vi "Cockpit_UDP_ receiver_IRISS_v2(2arms).vi"() -> ()   [LabVIEW 2016]
panel:
  in  "stop 2":bool
  out "deltaX 2":sgl
  out "data out 2":string
  out "length 2":i32
  out "deltaY 2":sgl
  out "deltaZ 2":sgl
  out "deltaRoll 2":sgl
  out "gripper 2":sgl
  out "down_pedal 2":sgl format="%.2f"
  out "up_pedal 2":bool
  out "left_pedal 2":bool
  out "right_pedal 2":bool
  out "Waveform Chart 8":sgl(graph)
  out "Waveform Chart 7":sgl(graph)
  out "Waveform Chart 6":sgl(graph)
  out "Waveform Chart 5":sgl(graph)
  out "Waveform Chart 4":sgl(graph)
  out "Waveform Chart 3":sgl(graph)
  out "Waveform Chart 2":sgl(graph)
  out "Waveform Chart":sgl(graph)
  out "right_pedal":bool
  out "left_pedal":bool
  out "up_pedal":bool
  out "gripper":sgl
  out "down_pedal":sgl format="%.2f"
  out "deltaRoll":sgl
  out "deltaZ":sgl
  out "deltaY":sgl
  out "length":i32
  out "data out":string
  out "deltaX":sgl
  in  "stop":bool
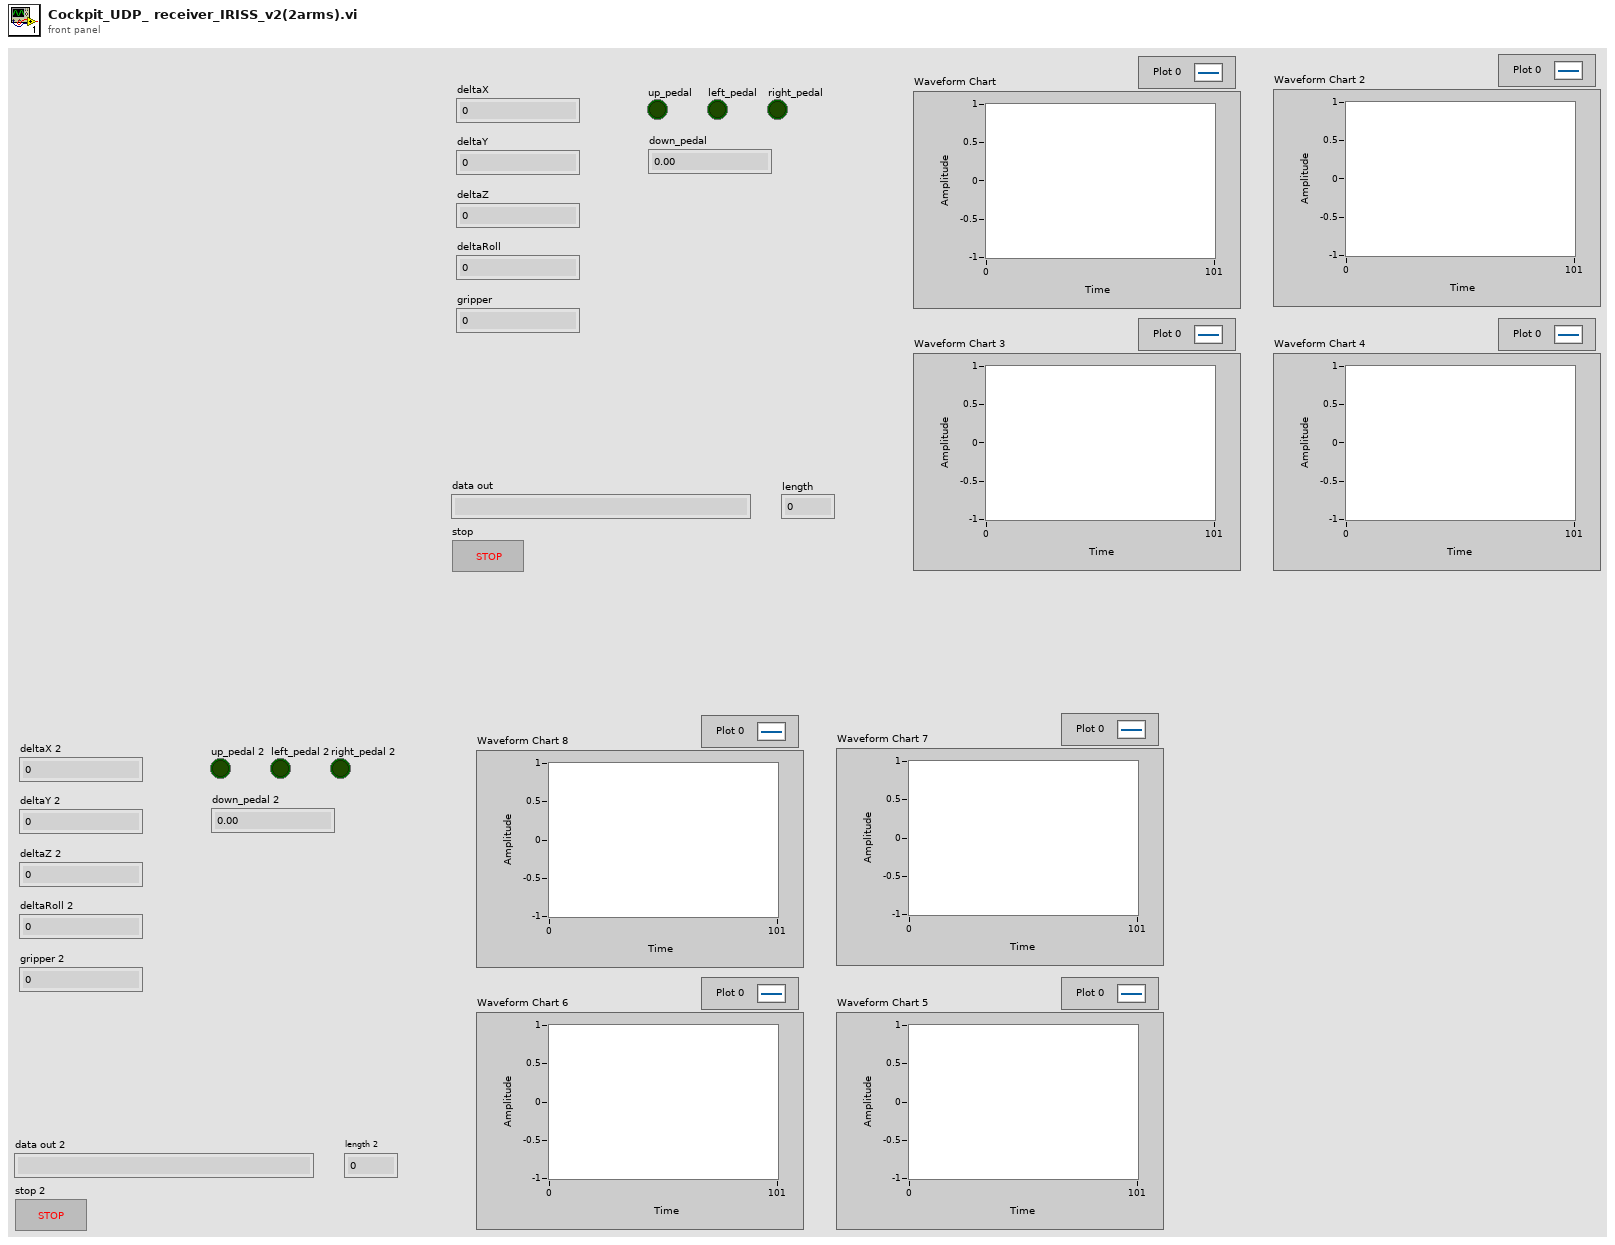
[diagram p1: front panel]
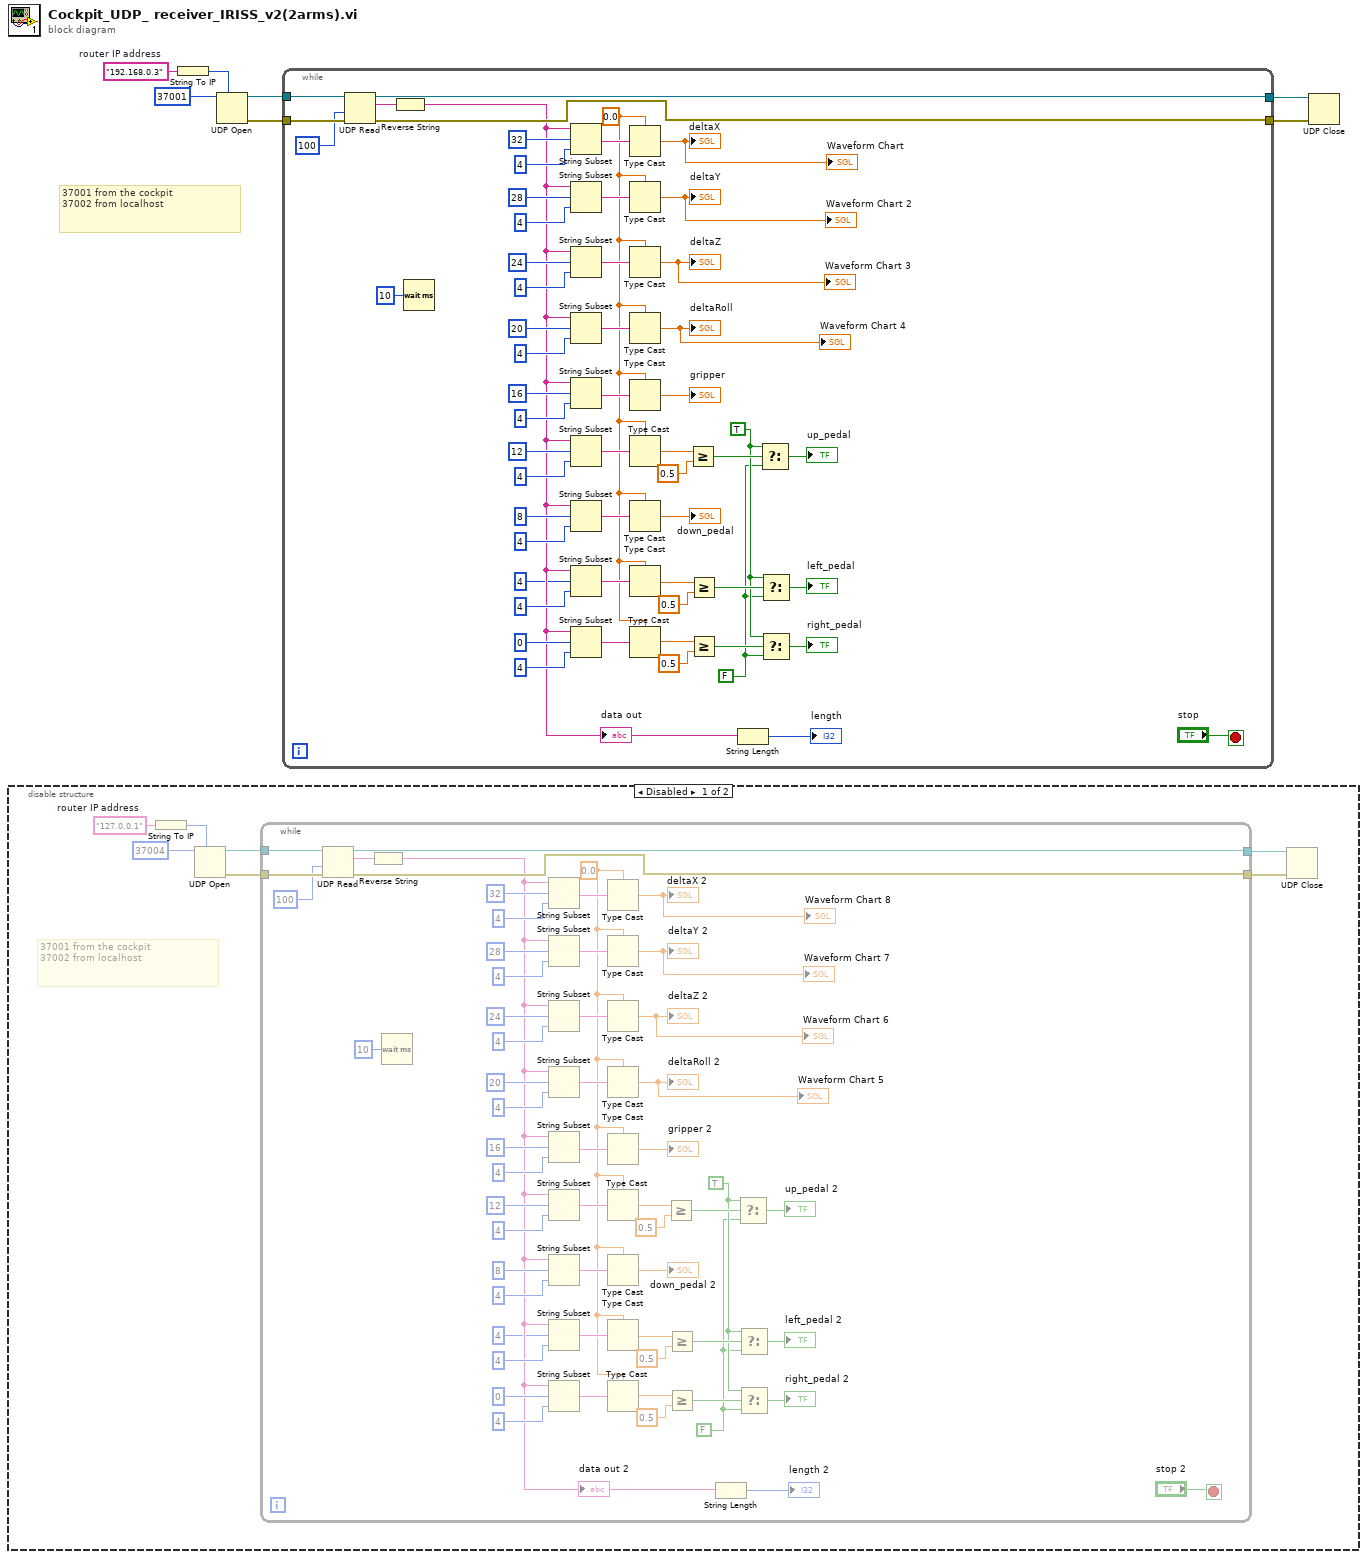
[diagram p0: block diagram]
diagram:
  w2 = "192.168.0.3"  # router IP address
  # "37001 from the cockpit\n37002 from localhost"
  n1 = disable-structure shown="Disabled" {
    frame Disabled {
      w9 = "127.0.0.1"  # router IP address
      # "37001 from the cockpit\n37002 from localhost"
      n2 = String To IP(1:w9) -> (0:w8:u32)
      n3 = UDP Open(7:w8, 11:u16 37004 ("port")) -> (port=w13:refnum<k16>, 0:w11:errorcluster)  [unwired: 3 in, 1 out]
      n4 = while {
        tunnel: w13 -> [w72]
        tunnel: [w70] -> w12
        tunnel: w11 -> [w41]
        tunnel: [w40] -> w10
        stop <- "stop 2" stop-if-true
        w25 = FALSE
        w26 = TRUE
        w36 = sgl 0.0
        n5 = UDP Read(connection ID=w72, timeout ms (25000)=100, 8:w41) -> (data out=w39:string, error out=w40:errorcluster, 3:w70:refnum<k16>)  [unwired: 1 in, 2 out]
        n6 = Reverse String(1:w39) -> (0:w38:string)
        "data out 2" <- w38
        n7 = Wait (ms)(milliseconds to wait=u32 10) -> ()  [unwired: 1 out]
        n8 = String Subset(string=w38, offset (0)=32, length (rest)=4 ("offset (0)")) -> (substring=w67:string)
        n9 = String Subset(string=w38, offset (0)=28, length (rest)=4 ("offset (0)")) -> (substring=w59:string)
        n10 = String Subset(string=w38, offset (0)=24, length (rest)=4 ("offset (0)")) -> (substring=w58:string)
        n11 = String Subset(string=w38, offset (0)=20, length (rest)=4 ("offset (0)")) -> (substring=w57:string)
        n12 = String Subset(string=w38, offset (0)=16, length (rest)=4 ("offset (0)")) -> (substring=w47:string)
        n13 = String Subset(string=w38, offset (0)=12, length (rest)=4 ("offset (0)")) -> (substring=w54:string)
        n14 = String Subset(string=w38, offset (0)=8, length (rest)=4 ("offset (0)")) -> (substring=w55:string)
        n15 = String Subset(string=w38, offset (0)=4, length (rest)=4 ("offset (0)")) -> (substring=w56:string)
        n16 = String Subset(string=w38, offset (0)=0, length (rest)=4 ("offset (0)")) -> (substring=w42:string)
        n17 = Type Cast(type=w36, x=w67) -> (*(type *) &x=→"deltaX 2" →"Waveform Chart 8":sgl)
        n18 = Type Cast(type=w36, x=w59) -> (*(type *) &x=→"deltaY 2" →"Waveform Chart 7":sgl)
        n19 = Type Cast(type=w36, x=w58) -> (*(type *) &x=→"deltaZ 2" →"Waveform Chart 6":sgl)
        n20 = Type Cast(type=w36, x=w57) -> (*(type *) &x=→"deltaRoll 2" →"Waveform Chart 5":sgl)
        n21 = Type Cast(type=w36, x=w47) -> (*(type *) &x=→"gripper 2":sgl)
        n22 = Type Cast(type=w36, x=w54) -> (*(type *) &x=w33:sgl)
        n23 = Type Cast(type=w36, x=w55) -> (*(type *) &x=→"down_pedal 2":sgl)
        n24 = Type Cast(type=w36, x=w56) -> (*(type *) &x=w27:sgl)
        n25 = Type Cast(type=w36, x=w42) -> (*(type *) &x=w28:sgl)
        n26 = Greater Or Equal?(x=w33, y=sgl 0.5) -> (x >= y?=w35:bool)
        n27 = Greater Or Equal?(x=w27, y=sgl 0.5) -> (x >= y?=w31:bool)
        n28 = Greater Or Equal?(x=w28, y=sgl 0.5) -> (x >= y?=w30:bool)
        n29 = String Length(string=w38) -> (length=→"length 2":i32)
        n30 = Select(t=w26, s=w35, f=w25) -> (s? t:f=→"up_pedal 2":bool)
        n31 = Select(t=w26, s=w31, f=w25) -> (s? t:f=→"left_pedal 2":bool)
        n32 = Select(t=w26, s=w30, f=w25) -> (s? t:f=→"right_pedal 2":bool)
      }
      n33 = UDP Close(connection ID=w12, 8:w10) -> ()  [unwired: 2 out]
    }
    frame Enabled {
    }
  }
  n34 = String To IP(1:w2) -> (0:w1:u32)
  n35 = UDP Open(7:w1, 11:u16 37001 ("port")) -> (port=w6:refnum<k16>, 0:w4:errorcluster)  [unwired: 3 in, 1 out]
  n36 = while {
    tunnel: w6 -> [w130]
    tunnel: [w128] -> w5
    tunnel: w4 -> [w99]
    tunnel: [w98] -> w3
    stop <- "stop" stop-if-true
    w83 = FALSE
    w84 = TRUE
    w94 = sgl 0.0
    n37 = UDP Read(connection ID=w130, timeout ms (25000)=100, 8:w99) -> (data out=w97:string, error out=w98:errorcluster, 3:w128:refnum<k16>)  [unwired: 1 in, 2 out]
    n38 = Reverse String(1:w97) -> (0:w96:string)
    "data out" <- w96
    n39 = Wait (ms)(milliseconds to wait=u32 10) -> ()  [unwired: 1 out]
    n40 = String Subset(string=w96, offset (0)=32, length (rest)=4 ("offset (0)")) -> (substring=w125:string)
    n41 = String Subset(string=w96, offset (0)=28, length (rest)=4 ("offset (0)")) -> (substring=w117:string)
    n42 = String Subset(string=w96, offset (0)=24, length (rest)=4 ("offset (0)")) -> (substring=w116:string)
    n43 = String Subset(string=w96, offset (0)=20, length (rest)=4 ("offset (0)")) -> (substring=w115:string)
    n44 = String Subset(string=w96, offset (0)=16, length (rest)=4 ("offset (0)")) -> (substring=w105:string)
    n45 = String Subset(string=w96, offset (0)=12, length (rest)=4 ("offset (0)")) -> (substring=w112:string)
    n46 = String Subset(string=w96, offset (0)=8, length (rest)=4 ("offset (0)")) -> (substring=w113:string)
    n47 = String Subset(string=w96, offset (0)=4, length (rest)=4 ("offset (0)")) -> (substring=w114:string)
    n48 = String Subset(string=w96, offset (0)=0, length (rest)=4 ("offset (0)")) -> (substring=w100:string)
    n49 = Type Cast(type=w94, x=w125) -> (*(type *) &x=→"deltaX" →"Waveform Chart":sgl)
    n50 = Type Cast(type=w94, x=w117) -> (*(type *) &x=→"deltaY" →"Waveform Chart 2":sgl)
    n51 = Type Cast(type=w94, x=w116) -> (*(type *) &x=→"deltaZ" →"Waveform Chart 3":sgl)
    n52 = Type Cast(type=w94, x=w115) -> (*(type *) &x=→"deltaRoll" →"Waveform Chart 4":sgl)
    n53 = Type Cast(type=w94, x=w105) -> (*(type *) &x=→"gripper":sgl)
    n54 = Type Cast(type=w94, x=w112) -> (*(type *) &x=w91:sgl)
    n55 = Type Cast(type=w94, x=w113) -> (*(type *) &x=→"down_pedal":sgl)
    n56 = Type Cast(type=w94, x=w114) -> (*(type *) &x=w85:sgl)
    n57 = Type Cast(type=w94, x=w100) -> (*(type *) &x=w86:sgl)
    n58 = Greater Or Equal?(x=w91, y=sgl 0.5) -> (x >= y?=w93:bool)
    n59 = Greater Or Equal?(x=w85, y=sgl 0.5) -> (x >= y?=w89:bool)
    n60 = Greater Or Equal?(x=w86, y=sgl 0.5) -> (x >= y?=w88:bool)
    n61 = String Length(string=w96) -> (length=→"length":i32)
    n62 = Select(t=w84, s=w93, f=w83) -> (s? t:f=→"up_pedal":bool)
    n63 = Select(t=w84, s=w89, f=w83) -> (s? t:f=→"left_pedal":bool)
    n64 = Select(t=w84, s=w88, f=w83) -> (s? t:f=→"right_pedal":bool)
  }
  n65 = UDP Close(connection ID=w5, 8:w3) -> ()  [unwired: 2 out]
